vi "Apply Gains And Decompose Color.vi"(8 "Error In":errorcluster, 10 "RGB Gains":T1, 11 "Color Box":u32(colorbox)) -> (0 "Error Out":errorcluster, 3 "Data":u8[](array[numeric]))   [LabVIEW 2021, in "Neopixel - Host.lvclass"]
uses:
  Neopixel - Host.lvclass
  Public/Controls/RGB Gains.ctl
  Neopixel - Host.lvclass/Neopixel - Host.ctl
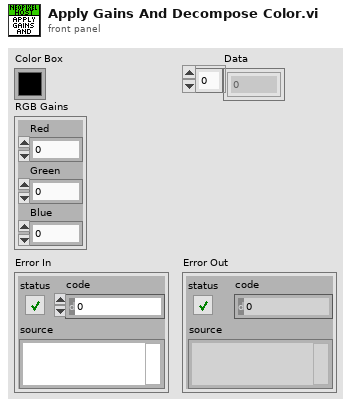
[diagram p1: front panel]
types:
  T1 = typedef "Neopixel - Host.lvclass/RGB Gains.ctl" = cluster{"Red":sgl, "Green":sgl, "Blue":sgl}
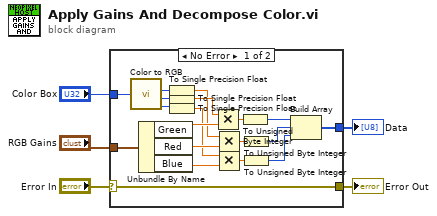
[diagram p0: block diagram]
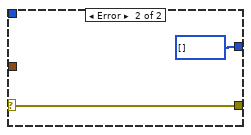
[diagram p2: hidden frame]
diagram:
  n1 = case shown="No Error" "Error In" {
    selector: "Error In" -> [w10 w26]
    tunnel: "RGB Gains" -> [w21 _]
    tunnel: "Color Box" -> [w11 _]
    tunnel: [w10 w26] -> w2
    tunnel: [w6 u8[] []] -> w1
    frame No Error {
      n2 = call <vilib>:"Color to RGB.vi"("Color"=w11) -> ("R"=w14:u8, "G"=w16:u8, "B"=w18:u8)  [unwired: 1 out]
      n3 = Unbundle By Name(w21) -> ("Green"=w22:sgl, "Red"=w23:sgl, "Blue"=w24:sgl)
      n4 = To Single Precision Float(number=w14) -> (single precision float=w15:sgl)
      n5 = To Single Precision Float(number=w16) -> (single precision float=w17:sgl)
      n6 = To Single Precision Float(number=w18) -> (single precision float=w19:sgl)
      n7 = Multiply(x=w17, y=w22) -> (x*y=w12:sgl)
      n8 = Multiply(x=w15, y=w23) -> (x*y=w13:sgl)
      n9 = Multiply(x=w19, y=w24) -> (x*y=w20:sgl)
      n10 = To Unsigned Byte Integer(number=w12) -> (unsigned 8bit integer=w9:u8)
      n11 = To Unsigned Byte Integer(number=w13) -> (unsigned 8bit integer=w8:u8)
      n12 = To Unsigned Byte Integer(number=w20) -> (unsigned 8bit integer=w7:u8)
      n13 = Build Array(w9, w8, w7) -> (w6:u8[])
    }
    frame Error {
    }
  }
  "Error Out" <- w2
  "Data" <- w1
